vi "XY Graph.vi"() -> ()   [LabVIEW 2023]
panel:
  out "XY Graph 2":cluster{"Y":dbl[], "Y":dbl[]}[](graph)
  out "XY Graph":cluster{"X":dbl[], "Y":dbl[]}[](graph)
  # "XY Graph"
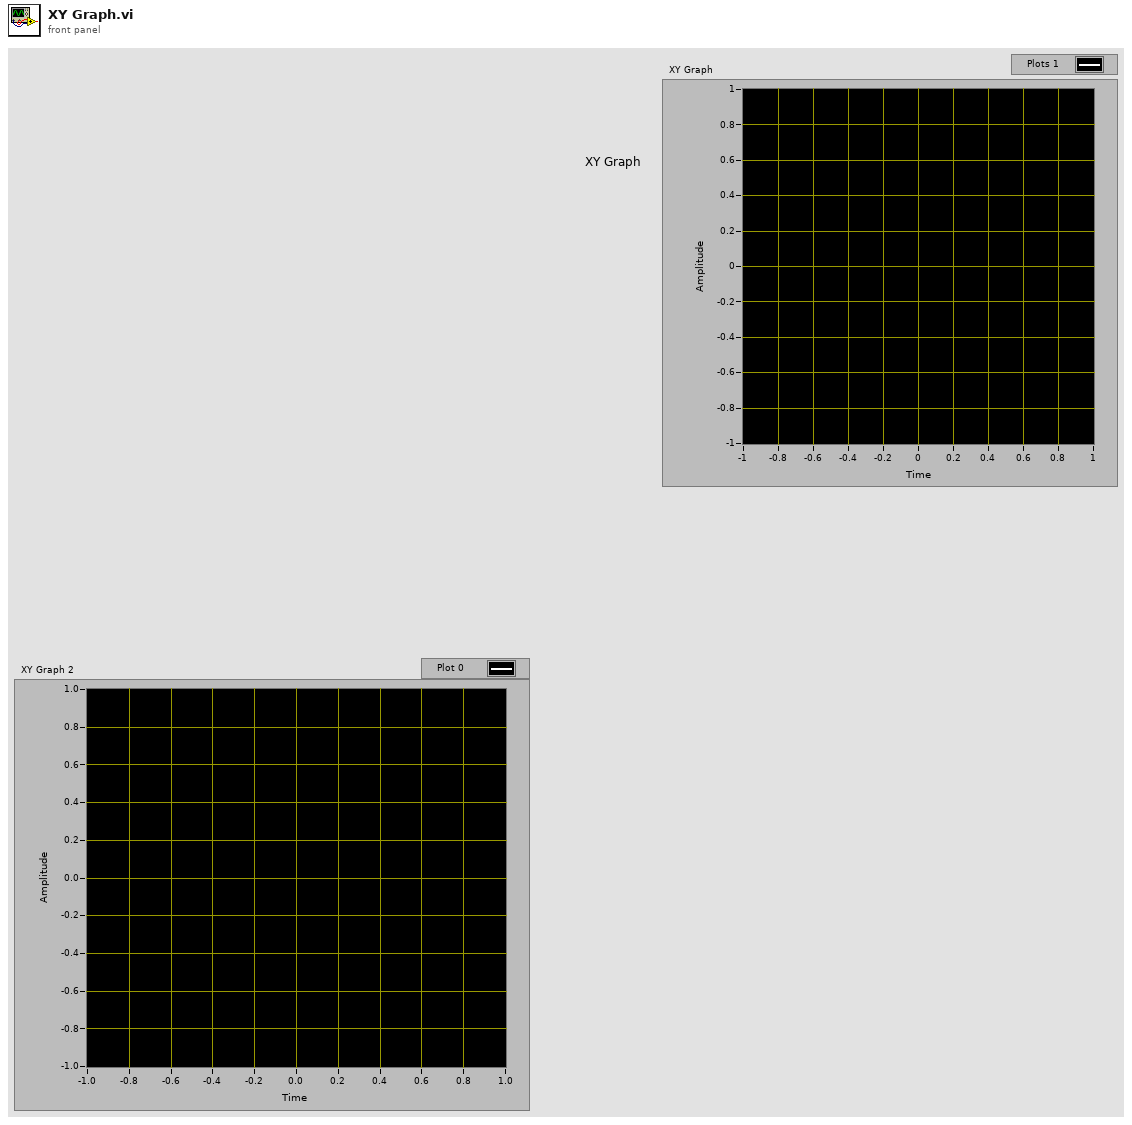
[diagram p1: front panel]
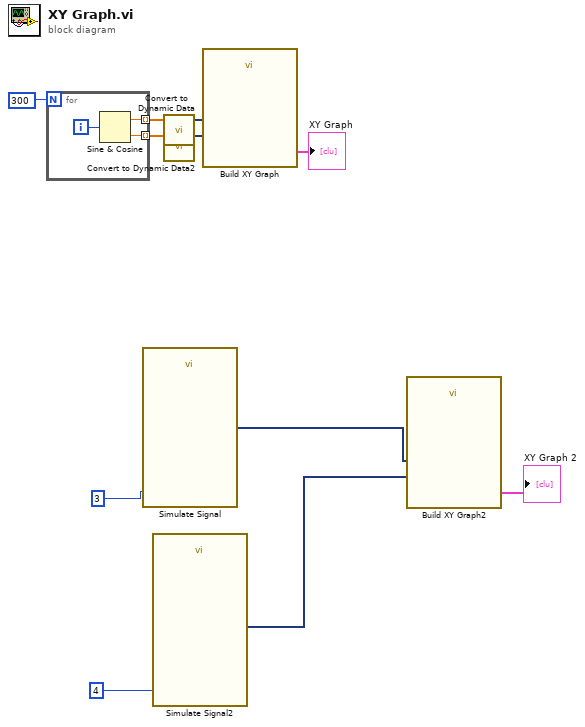
[diagram p0: block diagram]
diagram:
  n1 = for {
    N: 300 -> [_]
    tunnel: [w13] -> w10 mode=indexing
    tunnel: [w12] -> w8 mode=indexing
    i -> [w14]
    n2 = Sine & Cosine(0:w14) -> (1:w13:dbl, 2:w12:dbl)
  }
  n3 = call "Simulate Signal"("Frequency"=3) -> ("Sine"=w2:dynamicdata)  [unwired: 13 in, 1 out]
  n4 = call "Simulate Signal2"("Frequency"=4) -> ("Sine"=w1:dynamicdata)  [unwired: 13 in, 1 out]
  n5 = call "Convert to Dynamic Data"("Array"=w10) -> ("Dynamic Data Type"=w9:dynamicdata)  [unwired: 3 in]
  n6 = call "Convert to Dynamic Data2"("Array"=w8) -> ("Dynamic Data Type"=w7:dynamicdata)  [unwired: 3 in]
  n7 = call "Build XY Graph"("Y Input"=w7, "X Input"=w9) -> ("XY Graph"=→"XY Graph":cluster{"X":dbl[], "Y":dbl[]}[])  [unwired: 8 in, 1 out]
  n8 = call "Build XY Graph2"("Y Input"=w1, "X Input"=w2) -> ("XY Graph"=→"XY Graph 2":cluster{"X":dbl[], "Y":dbl[]}[])  [unwired: 8 in, 1 out]
